vi "Floor I32 at Zero.vi"(5 "Number":i32) -> (2 "Floored Number":i32)   [LabVIEW 2011]
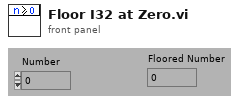
[diagram p1: front panel]
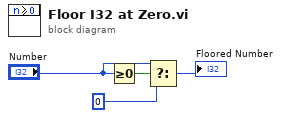
[diagram p0: block diagram]
diagram:
  n1 = Greater Or Equal To 0?(x="Number") -> (x >= 0?=w3:bool)
  n2 = Select(t="Number", s=w3, f=0) -> (s? t:f=→"Floored Number":i32)
